vi "Reset Supply.vi"(8 "error in":errorcluster, 11 "57XX in":refnum<class "57XX.lvclass">) -> (0 "error out":errorcluster, 3 "57XX out":refnum<class "57XX.lvclass">)   [LabVIEW 2019, in "57XX.lvlib" / "57XX.lvclass"]
uses:
  Library/57XX.lvclass
  Library/57XX.lvclass/57XX.ctl
  builds/Instruments/PowerSupply.lvlibp/Library/PowerSupply.lvclass
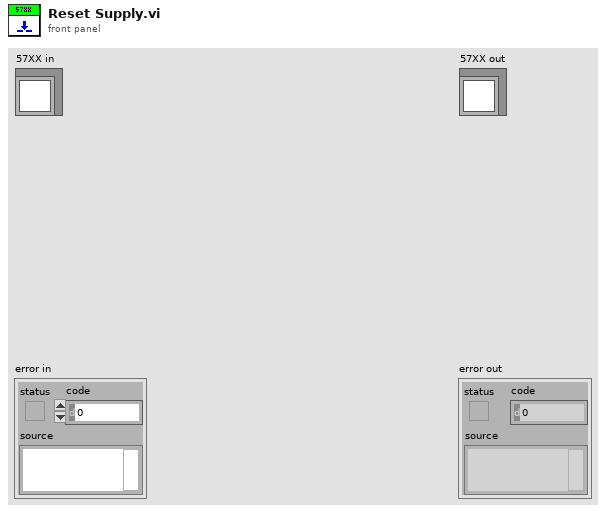
[diagram p1: front panel]
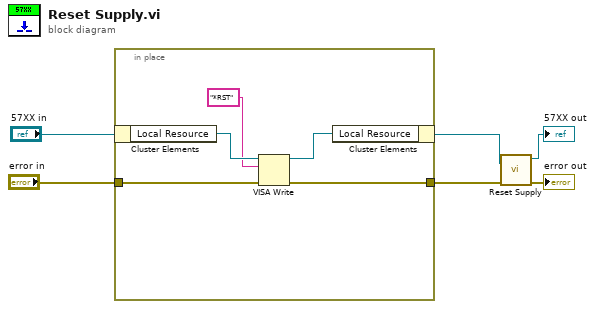
[diagram p0: block diagram]
diagram:
  n1 = in-place {
    in-place-border: "error in" -> [w8]
    in-place-border: [w7] -> w1
    n2 = in-place-cluster #1("57XX in") -> ("Local Resource"=w11:refnum<visa-resource-name>)
    n3 = VISA Write(VISA resource name=w11, write buffer="*RST", error in (no error)=w8) -> (VISA resource name out=w10:refnum<visa-resource-name>, error out=w7:errorcluster)  [unwired: 1 out]
    n4 = in-place-cluster #1("Local Resource"=w10) -> (w3:refnum<class "57XX.lvclass">)
  }
  n5 = call-parent "Reset Supply.vi"("error in"=w1, "PowerSupply in"=w3) -> ("error out"=→"error out":errorcluster, "PowerSupply out"=→"57XX out":refnum<class "57XX.lvclass">)  [unwired: 8 in]
